vi "Read Voltage.vi"(8 "error in (no error)":errorcluster, 11 "Driver In":refnum<class "Driver.lvclass">) -> (0 "error out":errorcluster, 2 "Voltage":dbl, 3 "Driver Out":refnum<class "Driver.lvclass">)   [LabVIEW 2020, in "Driver.lvclass"]
uses:
  Driver.lvclass
  Driver.lvclass/Driver.ctl
  Serial/Serial.lvclass/Serial.lvclass
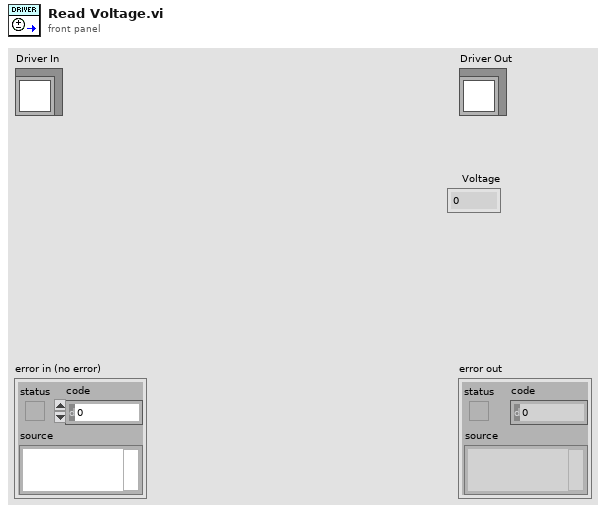
[diagram p1: front panel]
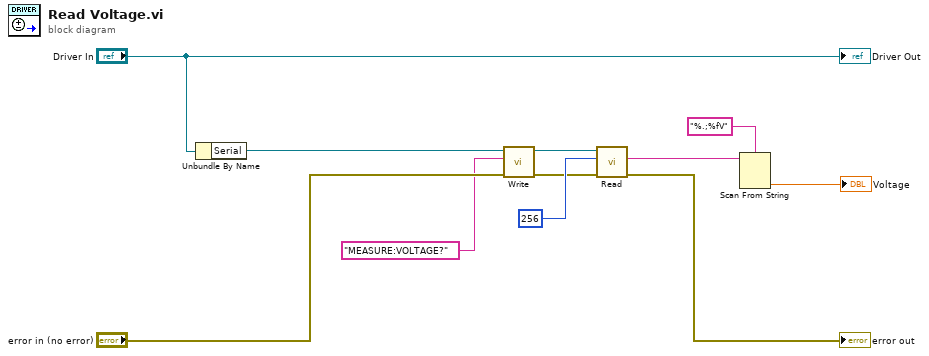
[diagram p0: block diagram]
diagram:
  n1 = Unbundle By Name("Driver In") -> ("Serial"=w10:refnum<class "Serial.lvclass">)
  n2 = call-dynamic "Write.vi"("error in (no error)"="error in (no error)", "write buffer"="MEASURE:VOLTAGE?", "Serial in"=w10) -> ("error out"=w2:errorcluster, "Serial out"=w1:refnum<class "Serial.lvclass">)  [unwired: 6 in, 1 out]
  n3 = call-dynamic "Read.vi"("error in (no error)"=w2, "byte count"=u32 256, "Serial in"=w1) -> ("error out"=→"error out":errorcluster, "read buffer"=w4:string)  [unwired: 6 in, 1 out]
  n4 = Scan From String(format string="%.;%fV", input string=w4) -> (output 1=→"Voltage":dbl)  [unwired: 3 in, 3 out]
  "Driver Out" <- "Driver In"
